vi "Error to String.vi"(2 "error in (no error)":errorcluster) -> (7 "message":string)   [LabVIEW 2019]
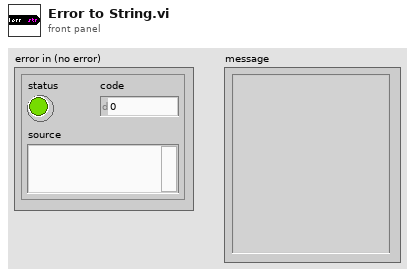
[diagram p1: front panel]
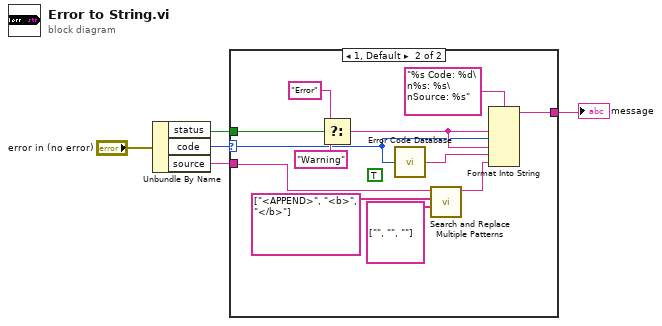
[diagram p0: block diagram]
diagram:
  n1 = Unbundle By Name("error in (no error)") -> ("status"=w4:bool, "code"=w3:i32, "source"=w1:string)
  n2 = case shown="1, Default" w3 {
    selector: w3 -> [_ w11]
    tunnel: w4 -> [_ w17]
    tunnel: [_ w12] -> w2
    tunnel: w1 -> [_ w8]
    frame 0 {
    }
    frame 1, Default {
      (unwired) TRUE ("replace all? (F)")
      n3 = Select(t="Error" ("format string"), s=w17, f="Warning" ("format string")) -> (s? t:f=w13:string)
      n4 = call <vilib>:"Error Code Database.vi"("Error Code"=w11) -> ("Error Text"=w10:string)
      n5 = call "Search and Replace Multiple Patterns.vi"("replace strings (\"\")"=string[] ["", "", ""] ("replace strings (\"\")"), "regular expressions"=string[] ["<APPEND>", "<b>", "</b>"] ("regular expression (\"\")"), "source"=w8) -> ("result string"=w9:string)  [unwired: 7 in, 1 out]
      n6 = Format Into String(format string="%s Code: %d\n%s: %s\nSource: %s", w13, w11, w13, w10, w9) -> (resulting string=w12:string)  [unwired: 2 in, 1 out]
    }
  }
  "message" <- w2
